vi "DmmPwr Simulator Scan.vi"() -> ()   [LabVIEW 2017]
doc: "This example shows how to configure a measurement and take multiple readings."
uses:
  DmmPwr Simulator.lvlib
panel:
  in  "Scan Dwelling (2 s)":dbl=2.0
  in  "Scan Steps (10)":u32=5
  in  "Scan Amplitude (30 V)":dbl=20.0
  in  "VISA resource name":refnum<visa-resource-name>="TCPIP::localhost::9997::SOCKET"
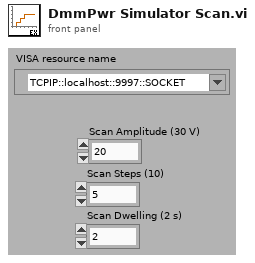
[diagram p1: front panel]
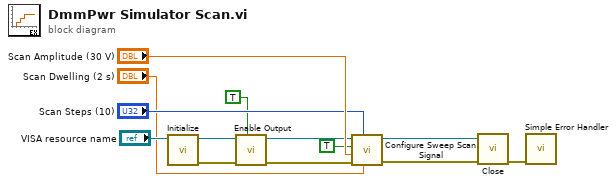
[diagram p0: block diagram]
diagram:
  n1 = call "Initialize.vi"("VISA resource name"="VISA resource name") -> ("error out"=w1:errorcluster, "VISA resource name out"=w6:refnum<visa-resource-name>)  [unwired: 9 in]
  n2 = call "Enable Output.vi"("Enable Output (F: Disable)"=TRUE, "error in (no error)"=w1, "VISA resource name"=w6) -> ("error out"=w2:errorcluster, "VISA resource name out"=w5:refnum<visa-resource-name>)  [unwired: 7 in]
  n3 = call "Configure Sweep Scan Signal.vi"("Scan Dwelling (2 s)"="Scan Dwelling (2 s)", "Scan Steps (10)"="Scan Steps (10)", "error in (no error)"=w2, "Scan Amplitude (30 V)"="Scan Amplitude (30 V)", "Wait? (Off)"=TRUE ("Wait?"), "VISA resource name"=w5) -> ("error out"=w3:errorcluster, "VISA resource name out"=w4:refnum<visa-resource-name>)  [unwired: 4 in]
  n4 = call "Close.vi"("error in (no error)"=w3, "VISA resource name"=w4) -> ("error out"=w13:errorcluster)  [unwired: 9 in]
  n5 = call <vilib>:"Simple Error Handler.vi"("error in (no error)"=w13) -> ()  [unwired: 4 in, 5 out]
